vi "FileIO.vi"() -> ()   [LabVIEW 2019]
panel:
  out "error out":errorcluster
  out "concatenated string":string
  in  "AngleInDeg":dbl
  in  "fileOut":path
  in  "error in":errorcluster
  in  "FileIn":path
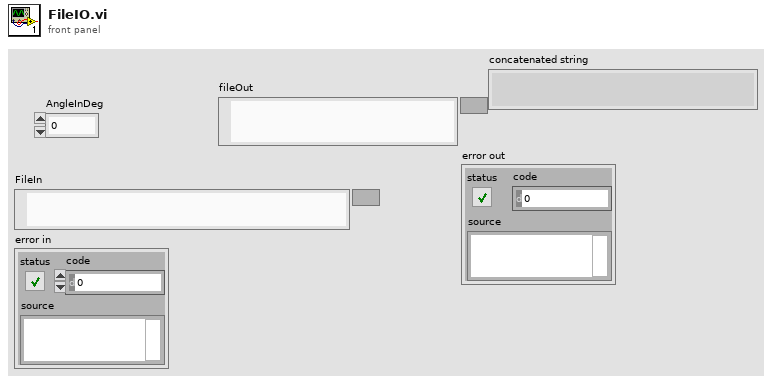
[diagram p1: front panel]
types:
  T1 = enum16{"open", "replace", "create", "open or create", "replace or create", "replace or create with confirmation"}
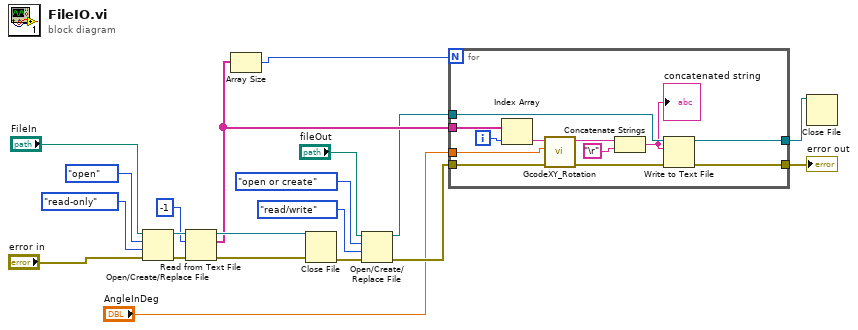
[diagram p0: block diagram]
diagram:
  n1 = Open/Create/Replace File(file path (use dialog)="FileIn", error in="error in", operation (0:open)=T1."open", access (0:read/write)=enum16{"read/write", "read-only", "write-only"}."read-only") -> (refnum out=w15:refnum<file>, error out=w16:errorcluster)  [unwired: 2 in, 1 out]
  n2 = Read from Text File(file (use dialog)=w15, count=-1, error in=w16) -> (refnum out=w13:refnum<file>, text=w11:string[], error out=w14:errorcluster)  [unwired: 1 in, 1 out]
  n3 = Array Size(array=w11) -> (size(s)=w10:i32)
  n4 = Close File(refnum=w13, error in=w14) -> (error out=w1:errorcluster)  [unwired: 1 out]
  n5 = Open/Create/Replace File(file path (use dialog)="fileOut", error in=w1, operation (0:open)=T1."open or create", access (0:read/write)=enum16{"read/write", "read-only", "write-only"}."read/write") -> (refnum out=w5:refnum<file>, error out=w6:errorcluster)  [unwired: 2 in, 1 out]
  n6 = for {
    N: w10 -> [_]
    tunnel: w11 -> [w32]
    tunnel: w6 -> [w22]
    tunnel: w5 -> [w28]
    tunnel: [w27] -> w4
    tunnel: [w26] -> w3
    tunnel: "AngleInDeg" -> [w23]
    i -> [w31]
    n7 = Index Array(array=w32, index=w31) -> (element=w30:string)
    n8 = call "GcodeXY_Rotation.vi"("error in"=w22, "AngleInDeg"=w23, "GCodeIn"=w30) -> ("error out 2"=w21:errorcluster, "GCodeOut"=w29:string)  [unwired: 3 in]
    n9 = Concatenate Strings(w29, "\r") -> (w24:string)
    "concatenated string" <- w24
    n10 = Write to Text File(file (use dialog)=w28, text=w24, error in=w21) -> (refnum out=w26:refnum<file>, error out=w27:errorcluster)  [unwired: 1 in, 1 out]
  }
  "error out" <- w4
  n11 = Close File(refnum=w3) -> ()  [unwired: 1 in, 2 out]
